vi "UpdateProject.vi"() -> ()   [LabVIEW 2020]
panel:
  in  "C++ Template":string="_scripts\\BlankProjects\\2023\\C++"
  in  "Java Template":string="_scripts\\BlankProjects\\2023\\Java"
  in  "C++ Root":string="C++"
  in  "Java Root":string="Java"
  out "Project Root":path
  # "Config"
  # "Warning! This VI will make copies of files and delete files on disk. Do not use this VI unless you know what you are doing!"
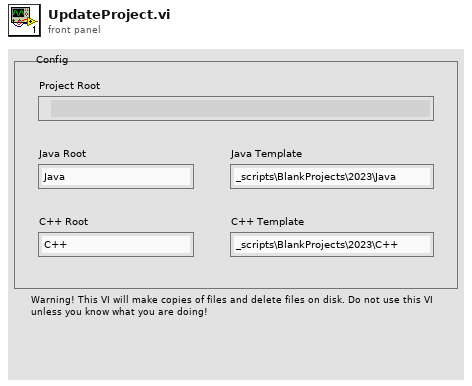
[diagram p1: front panel]
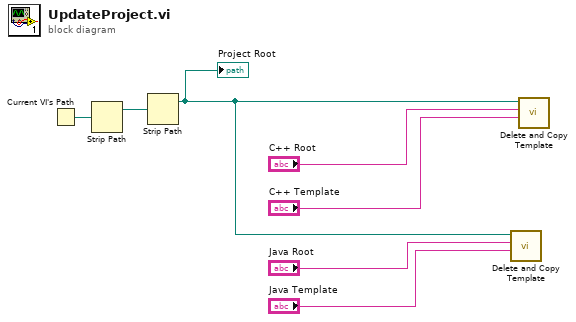
[diagram p0: block diagram]
diagram:
  n1 = Current VI's Path() -> (path=w7:path)
  n2 = Strip Path(path=w7) -> (stripped path=w6:path)  [unwired: 1 out]
  n3 = Strip Path(path=w6) -> (stripped path=w3:path)  [unwired: 1 out]
  "Project Root" <- w3
  n4 = call "Delete and Copy Template.vi"("Code Template"="Java Template", "Code Root"="Java Root", "Project Root"=w3) -> ()  [unwired: 9 in]
  n5 = call "Delete and Copy Template.vi"("Code Template"="C++ Template", "Code Root"="C++ Root", "Project Root"=w3) -> ()  [unwired: 9 in]
